vi "_Remote BlockUpdate.vi"(4 "error in":errorcluster, 6 "Filter (T)":bool=TRUE, 7 "Running":bool) -> (0 "error out":errorcluster)   [LabVIEW 2015]
uses:
  Type/_RT Active Ch.ctl
  Type/_RT Command.ctl
  Configuration/_Global Configuration.vi
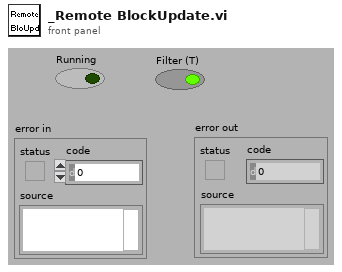
[diagram p1: front panel]
types:
  T1 = typedef "_RT Active Ch.ctl" = cluster{"Start":i32, "Step":i32, "ChID":i32}
  T2 = typedef "_Lens Property.ctl" = cluster{"Scan Type":u8, "Scans":i32, "Time 1":dbl, "Time 2":dbl, "Value 1":dbl, "Value 2":dbl, "Step Size":dbl}
  T3 = typedef "_Mass Range Property.ctl" = cluster{"Start":dbl, "Stop":dbl, "Step Size":dbl, "Steps":i32, "Dwell":dbl, "Parameters":T4[], "Res":T5}
  T4 = typedef "_Mass Range Parameters.ctl" = cluster{"Name":string, "Ch#":u8, "StartV":dbl, "StopV":dbl, "StepV":dbl, "Index":u8}
  T5 = typedef "_RT Res Type.ctl" = u16
  T6 = typedef "_Run Mode.ctl" = enum16{"MRM (Q1/Q2)", "Q1 Scan", "Q1 SRM", "Q2 Scan", "Q2 SRM", "Product Scan", "Precursor Scan", "Neutral Loss", "Neutral Gain"}
  T7 = cluster{"Lenses":T2[], "Mass Ranges":T3[], "Acquire":bool, "MCA":bool, "Q1DC EN":bool, "Q1 POL":bool, "Q3 POL":bool, "Q1 RF  EN":bool, "Averaging":bool, "Log Scale":bool, "CPS":bool, "Unit":bool, "Data Path":path, "Run Mode":T6, "Fixed Mass (amu)":dbl, "Q3DC EN":bool, "Q3 RF  EN":bool, "Negative":bool}
  T8 = typedef "_RT Instrument 2.ctl" = cluster{"Table":T9[], "Instrument":string[]}
  T9 = typedef "_RT Configuration 2.ctl" = cluster{"Name":string, "Ch#":u8, "Min":dbl, "Max":dbl, "Def+":dbl, "Def-":dbl, "Offset":dbl, "Slope":dbl, "Type":u8, "Description":string, "SettleT":dbl}
  T10 = typedef "_RT Command.ctl" = enum16{"Start", "Stop", "Runtime Update", "Get Data", "Get Info", "Get Status", "Get Param", "Get Config", "Get Table", "Read ADC", "Set Oscillator", "Update Config", "Update Table", "Set All Pol", "Set Pol and DC", "Set Max Mass", "Toggle RP", "Toggle EL", "Set PIC", "Initialize Turbo", "Send Turbo Comm", "Close Turbo", "P1", "P2", "P3", "Send Serial", "Set LC Out", "Get LC In", "Read VAC", "Test Table", "Toggle Power", "Get Startup", "Set Startup", "Get ADC Table", "Set ADC Table", "Get Brief Status", "Get Detail Status", "Auxiliary Update", "Set CC Logics", "Set CC Input Logics", "Ignore Error"}
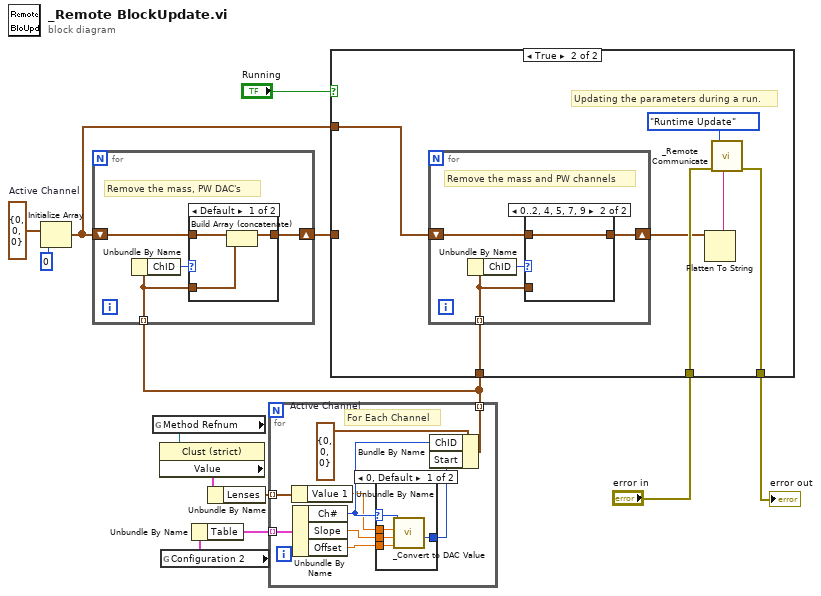
[diagram p0: block diagram]
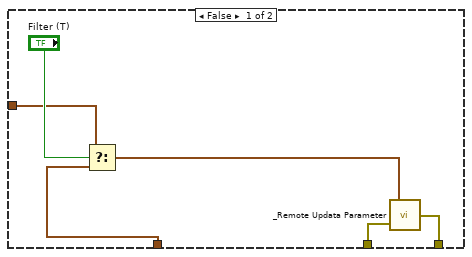
[diagram p3: hidden frame]
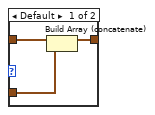
[diagram p4: hidden frame]
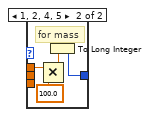
[diagram p5: hidden frame]
diagram:
  w4 = T1 {"Start"=0, "Step"=0, "ChID"=0}  # Active Channel
  n1 = Initialize Array(w4, 0 ("dimension size")) -> (w1:T1[])
  n2 = global read "_Global Configuration.vi" "Method Refnum"() -> (w10:refnum<vi>)
  n3 = property class="Clust (strict)"(reference=w10) -> ("Value"=w8:T7)  [unwired: 1 in, 2 out]
  n4 = global read "_Global Configuration.vi" "Configuration 2"() -> (w9:T8)
  n5 = Unbundle By Name(w9) -> ("Table"=w11:T9[])
  n6 = Unbundle By Name(w8) -> ("Lenses"=w7:T2[])
  n7 = for {
    tunnel: [w18] -> w3 mode=indexing
    tunnel: w11 -> [w16] mode=indexing
    tunnel: w7 -> [w15] mode=indexing
    w20 = T1 {"Start"=0, "Step"=0, "ChID"=0}  # Active Channel
    # "For Each Channel"
    n8 = Unbundle By Name(w15) -> ("Value 1"=w14:dbl)
    n9 = Unbundle By Name(w16) -> ("Ch#"=w17:u8, "Slope"=w22:dbl, "Offset"=w21:dbl)
    n10 = case shown="0, Default" w17 {
      selector: w17 -> [w23 _]
      tunnel: w14 -> [w27 w31]
      tunnel: w22 -> [w26 _]
      tunnel: w21 -> [w25 _]
      tunnel: [w24 w28] -> w19
      frame 0, Default {
        n11 = call "_Convert to DAC Value.vi"("Offset"=w25, "Slop"=w26, "Number"=w27, "Channel"=w23) -> ("DAC Value"=w24:i32)  [unwired: 2 in, 5 out]
      }
      frame 1, 2, 4, 5 {
        # "for mass"
        n12 = Multiply(x=w31, y=100.0) -> (x*y=w29:dbl)
        n13 = To Long Integer(number=w29) -> (32bit integer=w28:i32)
      }
    }
    n14 = Bundle By Name(cluster=w20, "ChID"=w17, "Start"=w19) -> (w18:T1)
  }
  n15 = for {
    shift-right: [w33] -> w2
    shift-left: w1 -> [w34]
    tunnel: w3 -> [w32] mode=indexing
    # "Remove the mass, PW DAC's"
    n16 = Unbundle By Name(w32) -> ("ChID"=w35:i32)
    n17 = case shown="Default" w35 {
      tunnel: [w36 w39] -> w33
      tunnel: w34 -> [w38 w39]
      tunnel: w32 -> [w37 _]
      frame Default {
        n18 = Build Array (concatenate)(w38, w37) -> (w36:T1[])
      }
      frame 0..2, 4, 5, 7, 9 {
      }
    }
  }
  n19 = case shown="True" "Running" {
    tunnel: "error in" -> [w41 w51]
    tunnel: [w42 w50] -> w12
    tunnel: w3 -> [w43 w48]
    tunnel: w2 -> [w44 _]
    tunnel: w1 -> [_ w46]
    frame False {
      n20 = Select(t=w44, s="Filter (T)", f=w43) -> (s? t:f=w40:T1[])
      n21 = call "_Remote Updata Parameter.vi"("error in"=w41, "Parameters"=w40) -> ("error out"=w42:errorcluster)
    }
    frame True {
      # "Updating the parameters during a run."
      n22 = for {
        shift-right: [w54] -> w47
        shift-left: w46 -> [w55]
        tunnel: w48 -> [w53] mode=indexing
        # "Remove the mass and PW channels"
        n23 = Unbundle By Name(w53) -> ("ChID"=w56:i32)
        n24 = case shown="0..2, 4, 5, 7, 9" w56 {
          tunnel: [w57 w60] -> w54
          tunnel: w55 -> [w59 w60]
          tunnel: w53 -> [w58 _]
          frame Default {
            n25 = Build Array (concatenate)(w59, w58) -> (w57:T1[])
          }
          frame 0..2, 4, 5, 7, 9 {
          }
        }
      }
      n26 = Flatten To String(anything=w47) -> (data string=w49:string)  [unwired: 1 in, 4 out]
      n27 = call "_Remote Communicate.vi"("String"=w49, "error in (no error)"=w51, "Command"=_RT_Command."Runtime Update") -> ("error out"=w50:errorcluster)  [unwired: 3 in, 3 out]
    }
  }
  "error out" <- w12
